vi "Time_to_MP.vi"(9 "sweep time tolerance (us)":dbl, 10 "freq_diff (Hz)":dbl, 11 "sweep time (ms)":dbl) -> (0 "Df":dbl, 1 "Dt":dbl, 2 "M":u32=65535, 3 "P":u32=65535, 4 "num":dbl, 5 "ctr":i32, 7 "T":dbl)   [LabVIEW 2016]
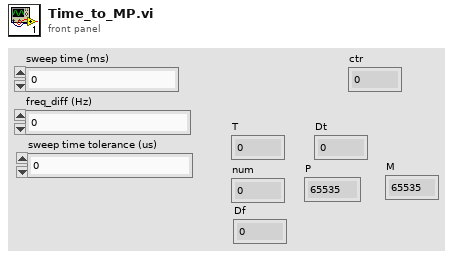
[diagram p1: front panel]
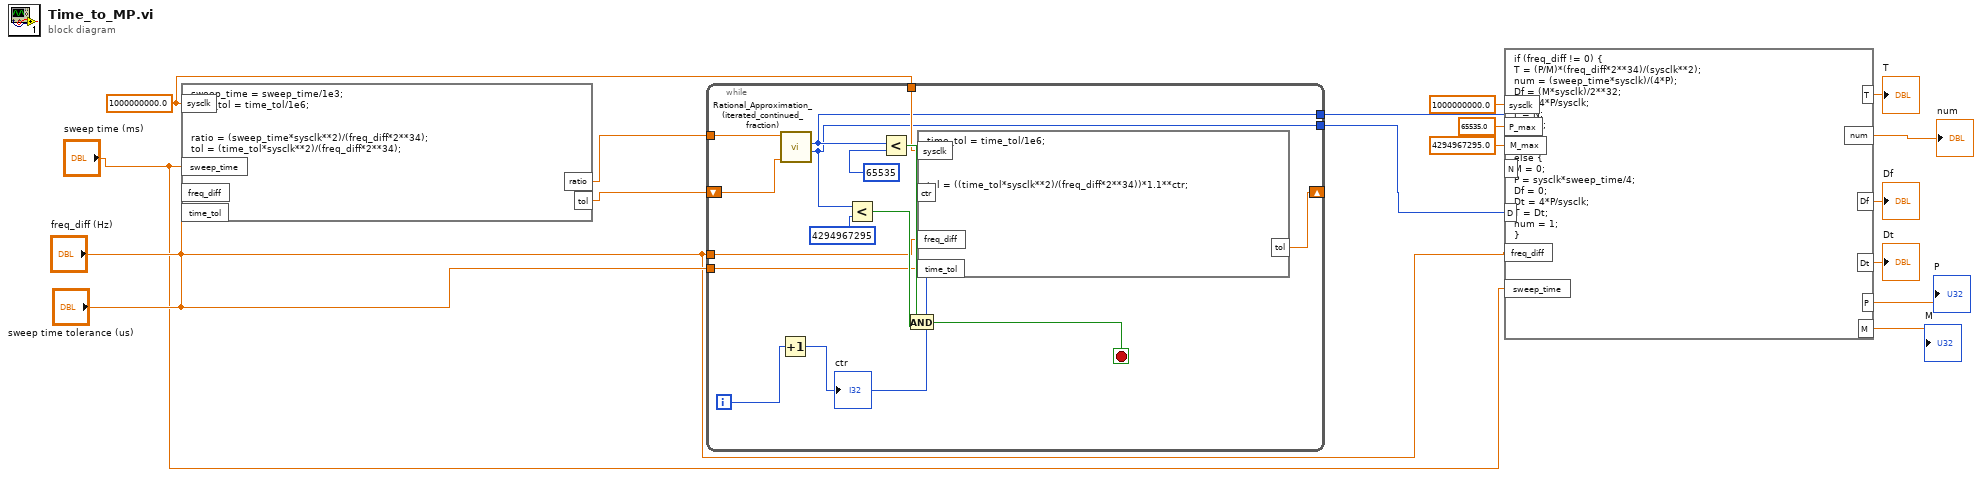
[diagram p0: block diagram]
diagram:
  w5 = 1000000000.0 ("input variable")
  n1 = formula code="sweep_time = sweep_time/1e3;\ntime_tol = time_tol/1e6;\n\n\nratio = (sweep_time*sysclk**2)/(freq_diff*2**34);\ntol = (time_tol*sysclk**2)/(freq_diff*2**34);"("sweep_time"="sweep time (ms)", "freq_diff"="freq_diff (Hz)", "time_tol"="sweep time tolerance (us)", "sysclk"=w5) -> ("ratio"=w8:dbl, "tol"=w7:dbl)
  n2 = while {
    tunnel: w8 -> [w32]
    shift-right: [w25] -> _
    shift-left: w7 -> [w30]
    tunnel: "freq_diff (Hz)" -> [w22]
    tunnel: "sweep time tolerance (us)" -> [w21]
    tunnel: w5 -> [w20]
    tunnel: [w19] -> w4
    tunnel: [w18] -> w3
    i -> [w23]
    stop <- w26 stop-if-true
    n3 = Increment(x=w23) -> (x+1=w24:i32)
    "ctr" <- w24
    n4 = call "Rational_Approximation_(iterated_continued_fraction).vi"("max error (1.0e-6)"=w30, "Orig floating point value"=w32) -> ("denominator"=w18:u32, "numerator"=w19:i32)  [unwired: 4 in, 4 out]
    n5 = Less?(x=w18, y=u32 4294967295) -> (x < y?=w27:bool)
    n6 = Less?(x=w19, y=65535) -> (x < y?=w28:bool)
    n7 = And(x=w28, y=w27) -> (x .and. y?=w26:bool)
    n8 = formula code="time_tol = time_tol/1e6;\n\n\n\ntol = ((time_tol*sysclk**2)/(freq_diff*2**34))*1.1**ctr;"("freq_diff"=w22, "time_tol"=w21, "sysclk"=w20, "ctr"=w24) -> ("tol"=w25:dbl)
  }
  n9 = formula code="if (freq_diff != 0) {\nT = (P/M)*(freq_diff*2**34)/(sysclk**2);\nnum = (sweep_time*sysclk)/(4*P);\nDf = (M*sysclk)/2**32;\nDt = 4*P/sysclk;\nP = N;\nM = D;\n}\n\nelse {\nM = 0;\nP = sysclk*sweep_time/4;\nDf = 0;\nDt = 4*P/sysclk;\nT = Dt;\nnum = 1;\n}"("N"=w4, "D"=w3, "sysclk"=1000000000.0 ("input variable"), "freq_diff"="freq_diff (Hz)", "sweep_time"="sweep time (ms)", "P_max"=65535.0 ("input variable"), "M_max"=4294967295.0 ("input variable")) -> ("T"=→"T":dbl, "num"=→"num":dbl, "Df"=→"Df":dbl, "Dt"=→"Dt":dbl, "P"=→"P":dbl, "M"=→"M":dbl)
